vi "Trace.vi"(0 "Execution Unit Implementation in":refnum<class "Execution Unit.lvclass">, 1 "message":string, 3 "error in (no error)":errorcluster) -> (7 "Execution Unit Implementation out":refnum<class "Execution Unit.lvclass">, 10 "error out":errorcluster)   [LabVIEW 2020, in "Communication Bus Template Engine.lvlib" / "Implementation.lvlib" / "Execution Unit.lvclass"]
uses:
  Execution Unit.lvclass
  Execution Unit.lvclass/Execution Unit.ctl
  <vilib>/Utility/SystemLogging/NI_SystemLogging.lvlib
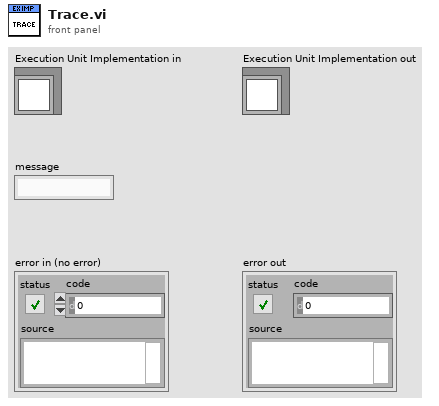
[diagram p1: front panel]
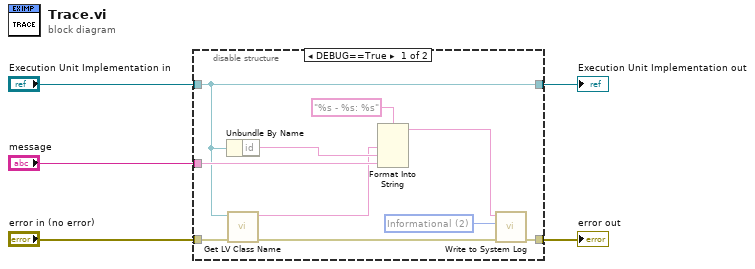
[diagram p0: block diagram]
diagram:
  n1 = disable-structure shown="DEBUG==True" {
    disable-tunnel: "message" -> [w15 _]
    disable-tunnel: [w12 w16] -> w4
    disable-tunnel: "error in (no error)" -> [w10 w16]
    disable-tunnel: "Execution Unit Implementation in" -> [w6 w17]
    disable-tunnel: [w6 w17] -> w1
    frame condition #0 {
      w13 = 2 items=["Error", "Warning", "Informational"] ("severity")
      n2 = Unbundle By Name(w6) -> ("id"=w8:string)
      n3 = call <vilib>:"Get LV Class Name.vi"("error in (no error)"=w10, "object"=w6) -> ("error out"=w9:errorcluster, "class name"=w7:string)  [unwired: 8 in]
      n4 = Format Into String(format string="%s - %s: %s", w7, w8, w15) -> (resulting string=w14:string)  [unwired: 2 in, 1 out]
      n5 = call <vilib>:"Write to System Log.vi"("error in (no error)"=w9, "severity"=w13, "message"=w14) -> ("error out"=w12:errorcluster)  [unwired: 8 in]
    }
    frame condition #1 (active) {
    }
  }
  "error out" <- w4
  "Execution Unit Implementation out" <- w1
